vi "Test MB 01 switches Module API.vi"() -> ()   [LabVIEW 2018]
doc: "MB 01 switches Module API Tester."
uses:
  MB 01 switches Module.lvlib
panel:
  out "trigger value?":bool
  in  "Read JIG trigger":bool
  in  "JIG Reset":bool
  in  "VISA resource name":refnum<visa-resource-name>="COM16"
  in  "MB01 Close":bool
  in  "5V enable":bool=TRUE
  in  "SC enable":bool
  in  "Array":bool[](array[boolean])=[FALSE, FALSE, FALSE, FALSE, FALSE, FALSE]
  in  "MB01_eMICs":bool
  in  "demux1_10(x6)_encode":T1(ring)
  in  "demux1-10":bool
  in  "MB01 Open":bool
  in  "Show Block Diagram":bool
  in  "Stop Module":bool
  in  "Start Module":bool
  in  "Hide Module Panel":bool
  in  "Show Module Panel":bool
  out "Status":string
  out "Module Running?":bool
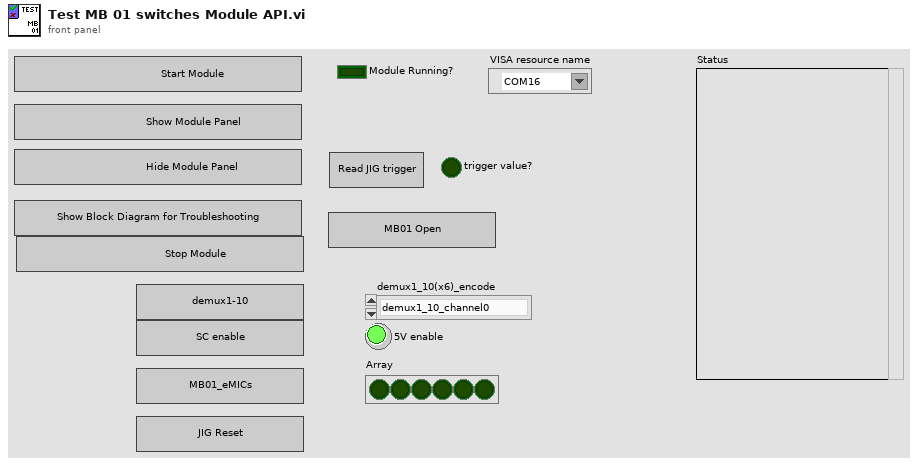
[diagram p1: front panel]
types:
  T1 = enum16{"demux1_10_channel0", "demux1_10_channel1", "demux1_10_channel2", "demux1_10_channel3", "demux1_10_channel4", "demux1_10_channel5", "demux1_10_channel6", "demux1_10_channel7", "demux1_10_channel8", "demux1_10_channel9", "demux1_10_channel10"}
  T2 = typedef "MB 01 switches Module.lvlib/Broadcast Events--cluster.ctl" = cluster{"Module Did Init":refnum<user-event>, "Status Updated":refnum<user-event>, "Error Reported":refnum<user-event>, "Module Did Stop":refnum<user-event>, "Update Module Execution Status":refnum<user-event>}
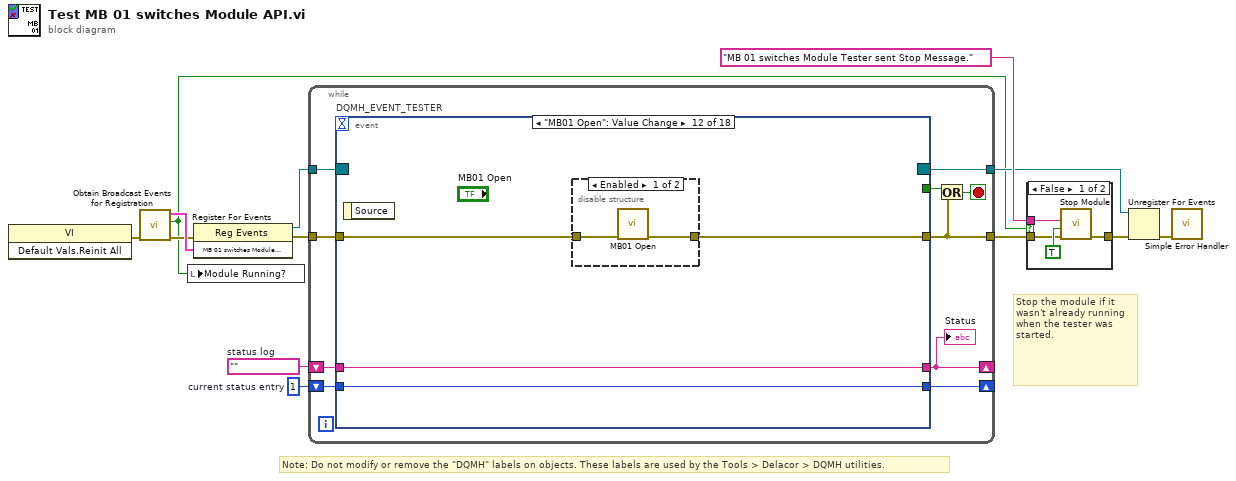
[diagram p0: block diagram]
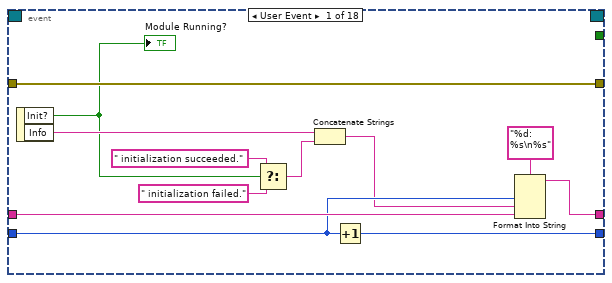
[diagram p3: hidden frame]
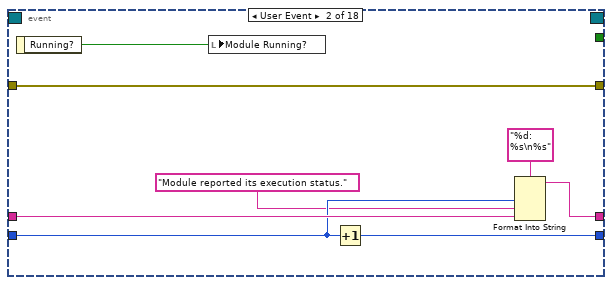
[diagram p4: hidden frame]
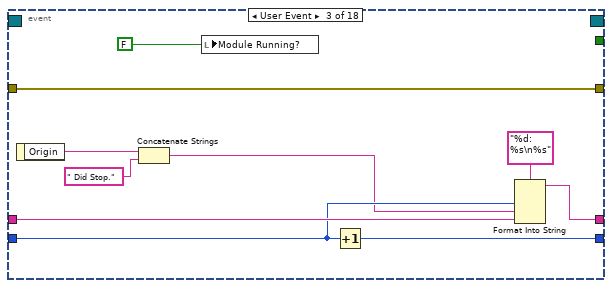
[diagram p5: hidden frame]
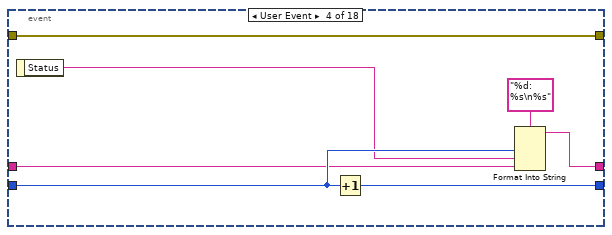
[diagram p6: hidden frame]
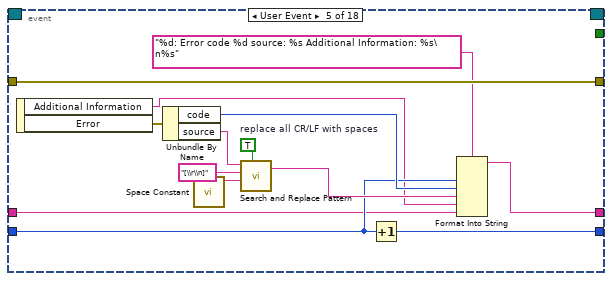
[diagram p7: hidden frame]
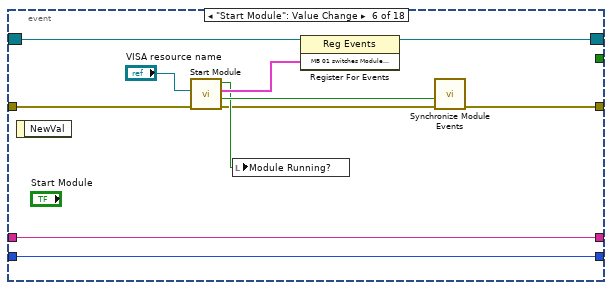
[diagram p8: hidden frame]
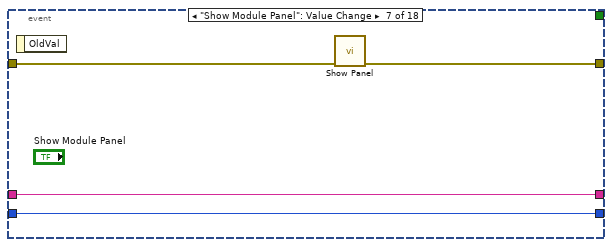
[diagram p9: hidden frame]
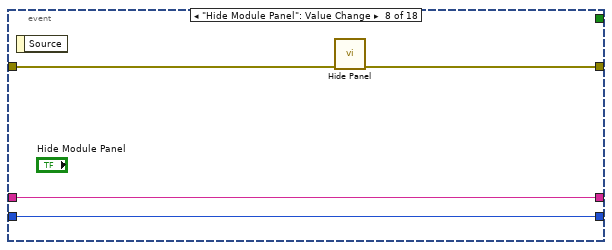
[diagram p10: hidden frame]
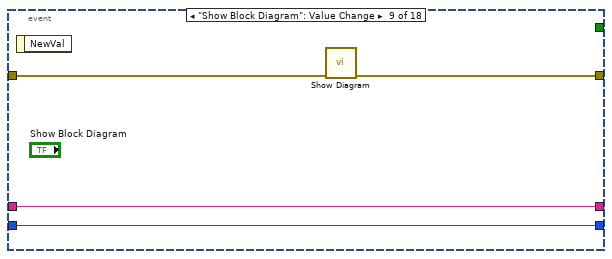
[diagram p11: hidden frame]
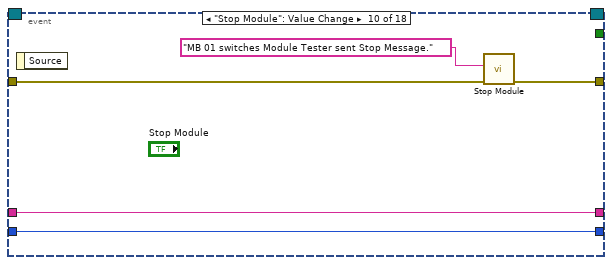
[diagram p12: hidden frame]
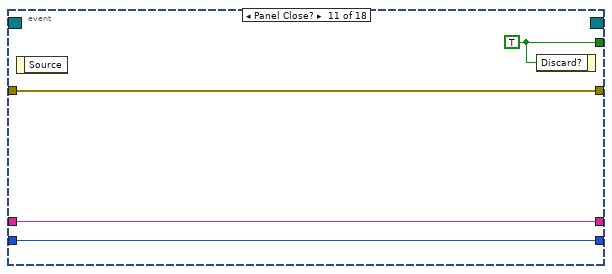
[diagram p13: hidden frame]
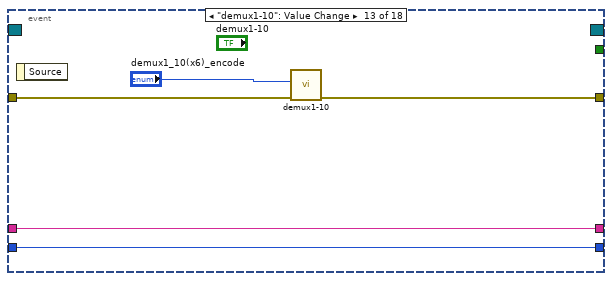
[diagram p15: hidden frame]
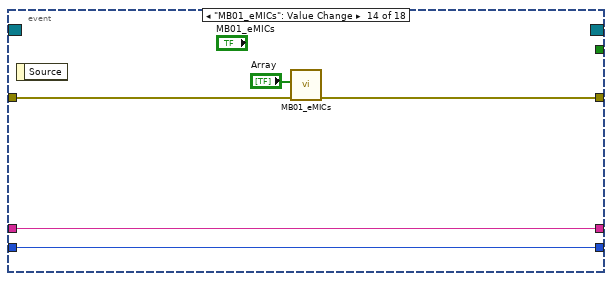
[diagram p16: hidden frame]
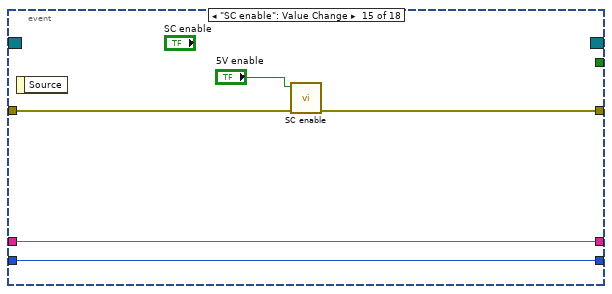
[diagram p17: hidden frame]
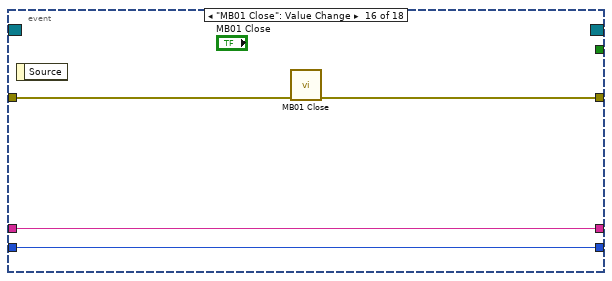
[diagram p18: hidden frame]
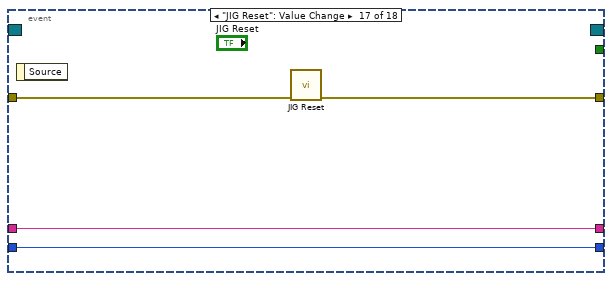
[diagram p19: hidden frame]
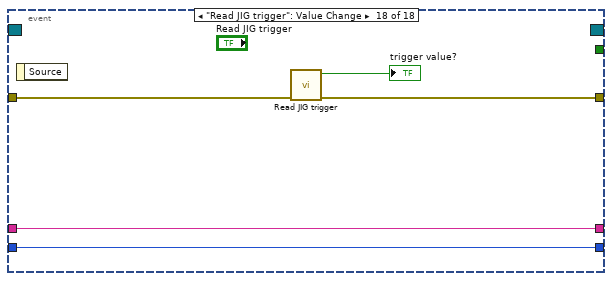
[diagram p20: hidden frame]
diagram:
  w10 = 1  # current status entry
  w11 = ""  # status log
  # "Stop the module if it wasn't already running when the tester was started."
  # "Note: Do not modify or remove the \"DQMH\" labels on objects. These labels are used by the Tools > Delacor > DQMH utilities."
  n1 = invoke class="VI" method="Default Vals.Reinit All"() -> (error out=w5:errorcluster)  [unwired: 3 in, 2 out]
  n2 = call "Obtain Broadcast Events for Registration.vi"("error in (no error)"=w5) -> ("error out"=w4:errorcluster, "Already running?"=w3:bool, "MB 01 switches Module Broadcast Events"=w8:T2)  [unwired: 8 in]
  n3 = local write "Module Running?"(w3) -> ()
  n4 = register-events(error in=w4, w8) -> (reference out=w7:refnum<event-registration>, error out=w9:errorcluster)  [unwired: 1 in]
  n5 = while {
    tunnel: w7 -> [w23]
    tunnel: [w14] -> w2
    shift-right: [w18] -> _
    shift-left: w11 -> [w20]
    shift-right: [w19] -> _
    shift-left: w10 -> [w21]
    tunnel: w9 -> [w16]
    tunnel: [w15] -> w6
    stop <- w17 stop-if-true
    n6 = event "DQMH_EVENT_TESTER" shown="[11] \"MB01 Open\": Value Change" {
      selector: w23 -> [_ _ _ _ _ w81 _ _ _ _ _ _ _ _ _ _ _ _]
      dyn-events: [_ _ _ _ _ w80 _ _ _ _ _ _ _ _ _ _ _ _] -> w15
      timeout: _ -> [_ _ _ _ _ _ _ _ _ _ _ _ _ _ _ _ _ _]
      tunnel: [_ _ _ _ _ _ _ _ _ _ w106 _ _ _ _ _ _ _] -> w22
      tunnel: [w35 w37 w44 w54 w74 w79 w89 w93 w94 w100 w103 w107 w115 w120 w125 w129 w133 w138] -> w14
      tunnel: w21 -> [w32 w41 w51 w57 w64 w84 w87 w91 w95 w101 w104 w108 w116 w121 w126 w130 w134 w139]
      tunnel: w20 -> [w33 w42 w52 w56 w62 w85 w88 w92 w96 w102 w105 w109 w117 w122 w127 w131 w135 w140]
      tunnel: [w30 w39 w49 w58 w65 w85 w88 w92 w96 w102 w105 w109 w117 w122 w127 w131 w135 w140] -> w18
      tunnel: [w31 w40 w50 w60 w63 w84 w87 w91 w95 w101 w104 w108 w116 w121 w126 w130 w134 w139] -> w19
      tunnel: w16 -> [w35 w37 w44 w54 w74 w78 w86 w90 w97 w98 w103 w110 w118 w123 w128 w132 w136 w141]
      event User Event {
        n7 = event-data() -> ("Init?"=w27:bool, "Info"=w29:string)  [unwired: 1 in]
        "Module Running?" <- w27
        n8 = Select(t=" initialization succeeded.", s=w27, f=" initialization failed.") -> (s? t:f=w24:string)
        n9 = Concatenate Strings(w29, w24) -> (w28:string)
        n10 = Increment(x=w32) -> (x+1=w31:i32)
        n11 = Format Into String(format string="%d: %s\n%s", w32, w28, w33) -> (resulting string=w30:string)  [unwired: 2 in, 1 out]
      }
      event User Event {
        n12 = event-data() -> ("Running?"=w36:bool)  [unwired: 1 in]
        n13 = local write "Module Running?"(w36) -> ()
        n14 = Increment(x=w41) -> (x+1=w40:i32)
        n15 = Format Into String(format string="%d: %s\n%s", w41, "Module reported its execution status.", w42) -> (resulting string=w39:string)  [unwired: 2 in, 1 out]
      }
      event User Event {
        n16 = event-data() -> ("Origin"=w48:string)  [unwired: 1 in]
        n17 = Concatenate Strings(w48, " Did Stop.") -> (w47:string)
        n18 = local write "Module Running?"(FALSE ("Module Did Init?")) -> ()
        n19 = Increment(x=w51) -> (x+1=w50:i32)
        n20 = Format Into String(format string="%d: %s\n%s", w51, w47, w52) -> (resulting string=w49:string)  [unwired: 2 in, 1 out]
      }
      event User Event {
        n21 = event-data() -> ("Status"=w55:string)  [unwired: 1 in]
        n22 = Increment(x=w57) -> (x+1=w60:i32)
        n23 = Format Into String(format string="%d: %s\n%s", w57, w55, w56) -> (resulting string=w58:string)  [unwired: 2 in, 1 out]
      }
      event User Event {
        w70 = TRUE  # replace all CR/LF with spaces
        n24 = event-data() -> ("Additional Information"=w61:string, "Error"=w66:errorcluster)  [unwired: 1 in]
        n25 = Unbundle By Name(w66) -> ("code"=w67:i32, "source"=w68:string)
        n26 = call <vilib>:"Space Constant.vi"() -> ("String"=w71:string)
        n27 = call <vilib>:"Search and Replace Pattern.vi"("string"=w68, "regular expression (\"\")"="[\\r\\n]" ("regular expression (\"\")"), "replace string (\"\")"=w71, "replace all? (F)"=w70) -> ("result string"=w69:string)  [unwired: 1 in, 1 out]
        n28 = Increment(x=w64) -> (x+1=w63:i32)
        n29 = Format Into String(format string="%d: Error code %d source: %s Additional Information: %s\n%s", w64, w67, w69, w61, w62) -> (resulting string=w65:string)  [unwired: 2 in, 1 out]
      }
      event "Start Module": Value Change {
        n30 = event-data() -> ()  [unwired: 1 in, 1 out]
        n31 = call "Start Module.vi"("error in (no error)"=w78, "COMport name"="VISA resource name") -> ("error out"=w75:errorcluster, "Wait for Event Sync?"=w83:bool, "MB 01 switches Module Broadcast Events"=w82:T2, "Module Was Already Running?"=w77:bool)  [unwired: 6 in]
        n32 = local write "Module Running?"(w77) -> ()
        n33 = register-events(reference=w81, w82) -> (reference out=w80:refnum<event-registration>)  [unwired: 1 in, 1 out]
        n34 = call "Synchronize Module Events.vi"("error in"=w75, "Wait for Event Sync?"=w83) -> ("error out"=w79:errorcluster)  [unwired: 9 in]
      }
      event "Show Module Panel": Value Change {
        n35 = event-data() -> ()  [unwired: 1 in, 1 out]
        n36 = call "Show Panel.vi"("error in (no error)"=w86) -> ("error out"=w89:errorcluster)  [unwired: 10 in]
      }
      event "Hide Module Panel": Value Change {
        n37 = event-data() -> ()  [unwired: 1 in, 1 out]
        n38 = call "Hide Panel.vi"("error in (no error)"=w90) -> ("error out"=w93:errorcluster)  [unwired: 10 in]
      }
      event "Show Block Diagram": Value Change {
        n39 = event-data() -> ()  [unwired: 1 in, 1 out]
        n40 = call "Show Diagram.vi"("error in (no error)"=w97) -> ("error out"=w94:errorcluster)  [unwired: 10 in]
      }
      event "Stop Module": Value Change {
        n41 = event-data() -> ()  [unwired: 1 in, 1 out]
        n42 = call "Stop Module.vi"("error in"=w98, "Origin"="MB 01 switches Module Tester sent Stop Message.") -> ("error out"=w100:errorcluster)  [unwired: 9 in]
      }
      event Panel Close? {
        w106 = TRUE ("Discard?")
        n43 = event-data() -> ()  [unwired: 1 in, 1 out]
        n44 = event-data("Discard?"=w106) -> ()  [unwired: 1 in, 1 out]
      }
      event "MB01 Open": Value Change {
        n45 = event-data() -> ()  [unwired: 1 in, 1 out]
        n46 = disable-structure shown="Enabled" {
          disable-tunnel: w110 -> [w112 w113]
          disable-tunnel: [w111 w113] -> w107
          frame Enabled {
            n47 = call "MB01 Open.vi"("error in"=w112) -> ("error out"=w111:errorcluster)  [unwired: 10 in]
          }
          frame Disabled {
          }
        }
      }
      event "demux1-10": Value Change {
        n48 = event-data() -> ()  [unwired: 1 in, 1 out]
        n49 = call "demux1-10.vi"("error in"=w118, "demux1_10(x6)_encode"="demux1_10(x6)_encode") -> ("error out"=w115:errorcluster)  [unwired: 9 in]
      }
      event "MB01_eMICs": Value Change {
        n50 = event-data() -> ()  [unwired: 1 in, 1 out]
        n51 = call "MB01_eMICs.vi"("error in"=w123, "Array"="Array") -> ("error out"=w120:errorcluster)  [unwired: 9 in]
      }
      event "SC enable": Value Change {
        n52 = event-data() -> ()  [unwired: 1 in, 1 out]
        n53 = call "SC enable.vi"("error in"=w128, "5V enable"="5V enable") -> ("error out"=w125:errorcluster)  [unwired: 9 in]
      }
      event "MB01 Close": Value Change {
        n54 = event-data() -> ()  [unwired: 1 in, 1 out]
        n55 = call "MB01 Close.vi"("error in"=w132) -> ("error out"=w129:errorcluster)  [unwired: 10 in]
      }
      event "JIG Reset": Value Change {
        n56 = event-data() -> ()  [unwired: 1 in, 1 out]
        n57 = call "JIG Reset.vi"("error in"=w136) -> ("error out"=w133:errorcluster)  [unwired: 10 in]
      }
      event "Read JIG trigger": Value Change {
        n58 = event-data() -> ()  [unwired: 1 in, 1 out]
        n59 = call "Read JIG trigger.vi"("error in"=w141) -> ("error out"=w138:errorcluster, "Trigger?"=→"trigger value?":bool)  [unwired: 8 in, 1 out]
      }
    }
    "Status" <- w18
    n60 = Or(x=w22, y=w14) -> (x .or. y?=w17:bool)
  }
  n61 = case shown="False" w3 {
    tunnel: [w145 w146] -> w13
    tunnel: "MB 01 switches Module Tester sent Stop Message." ("Origin") -> [w144 _]
    tunnel: w2 -> [w142 w146]
    frame False {
      n62 = call "Stop Module.vi"("error in"=w142, "Wait for Module to Stop? (F)"=TRUE ("Wait for Module to stop?"), "Origin"=w144) -> ("error out"=w145:errorcluster)  [unwired: 8 in]
    }
    frame True {
    }
  }
  n63 = Unregister For Events(event registration refnum=w6, error in=w13) -> (error out=w1:errorcluster)
  n64 = call <vilib>:"Simple Error Handler.vi"("error in (no error)"=w1) -> ()  [unwired: 4 in, 5 out]
